vi "增加角点.vi"(9 "原始角点坐标":cluster{"X":sgl, "Y":sgl}[](array[cluster]), 11 "Image In":T1) -> (1 "原始角点坐标 2":cluster{"X":sgl, "Y":sgl}[](array[cluster]), 3 "角点图":T1(plugin-control))   [LabVIEW 2018]
uses:
  <vilib>/vision/Image Controls.llb/IMAQ Image.ctl
  <vilib>/vision/NI_Vision_Development_Module.lvlib
panel:
  in  "角点的最小强度":i32
  in  "刷新按钮":bool
  in  "快进按钮":bool
  out "Corner Point Coordinates":cluster{"X":sgl, "Y":sgl}[](array[cluster])
  out "Image (duplicate)":T1
  in  "确定按钮":bool
  in  "停止角点增加":bool
  in  "操作类型":bool
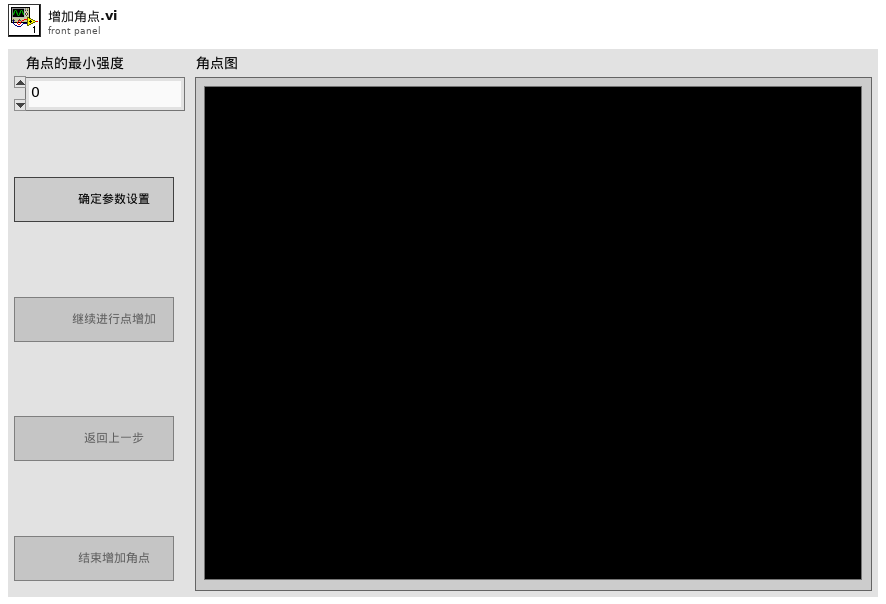
[diagram p1: front panel]
types:
  T1 = typedef "IMAQ Image.ctl" = refnum<image>
  T2 = enum8{"Enabled", "Disabled", "Disabled and Grayed Out"}
  T3 = typedef "IMAQ Rectangle" = cluster{"Left":i32, "Top":i32, "Right":i32, "Bottom":i32, "Rotation":dbl}
  T4 = typedef "ROI Descriptor" = cluster{"Global Rectangle":i32[], "Contours":cluster{"ID":enum32{"External", "Internal"}, "Type":u32, "Coordinates":i32[]}[]}
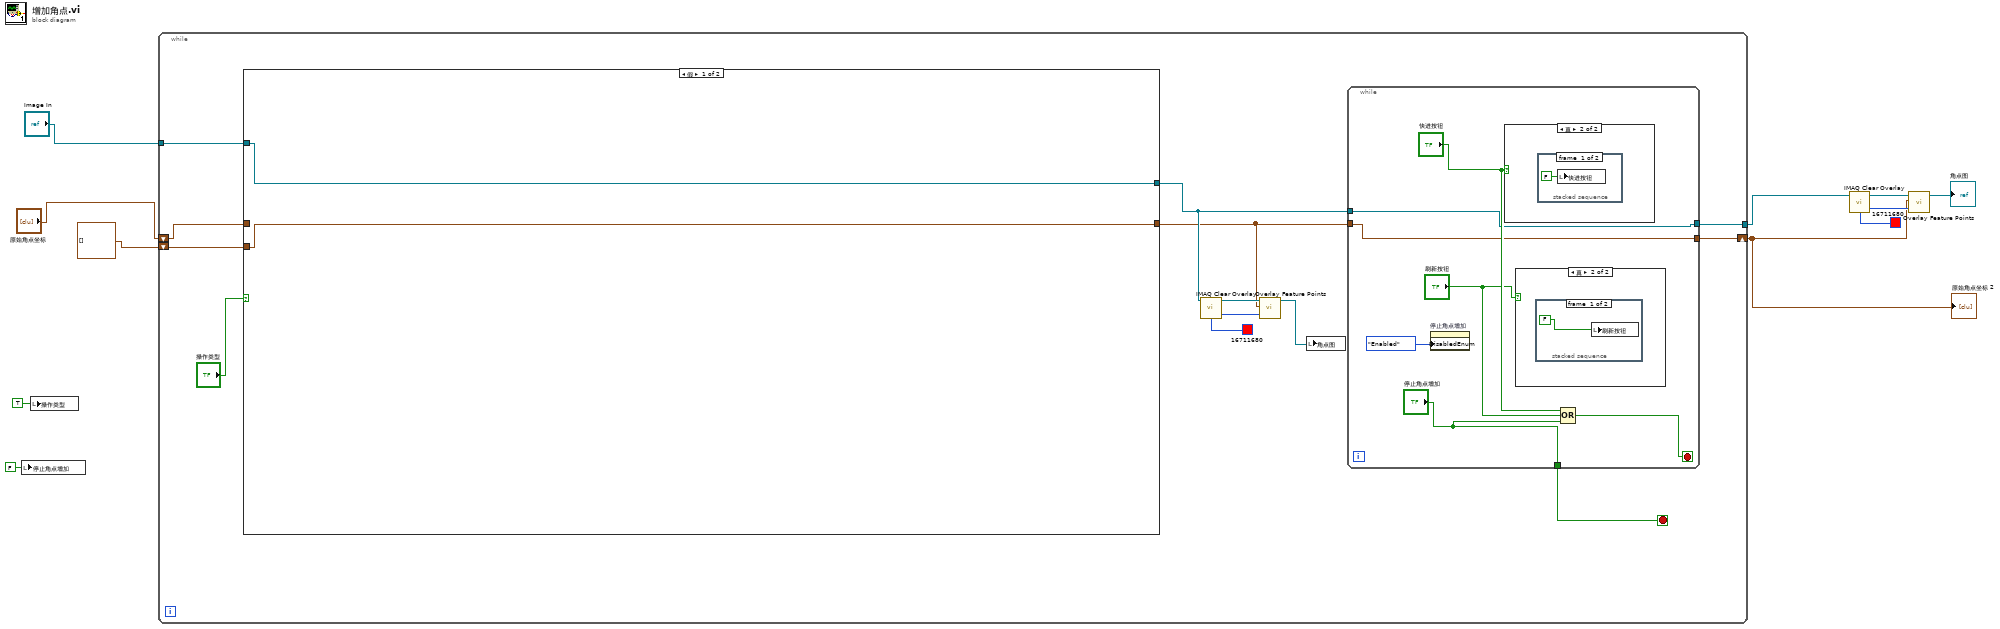
[diagram p0: block diagram]
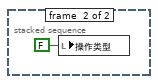
[diagram p3: hidden frame]
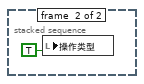
[diagram p5: hidden frame]
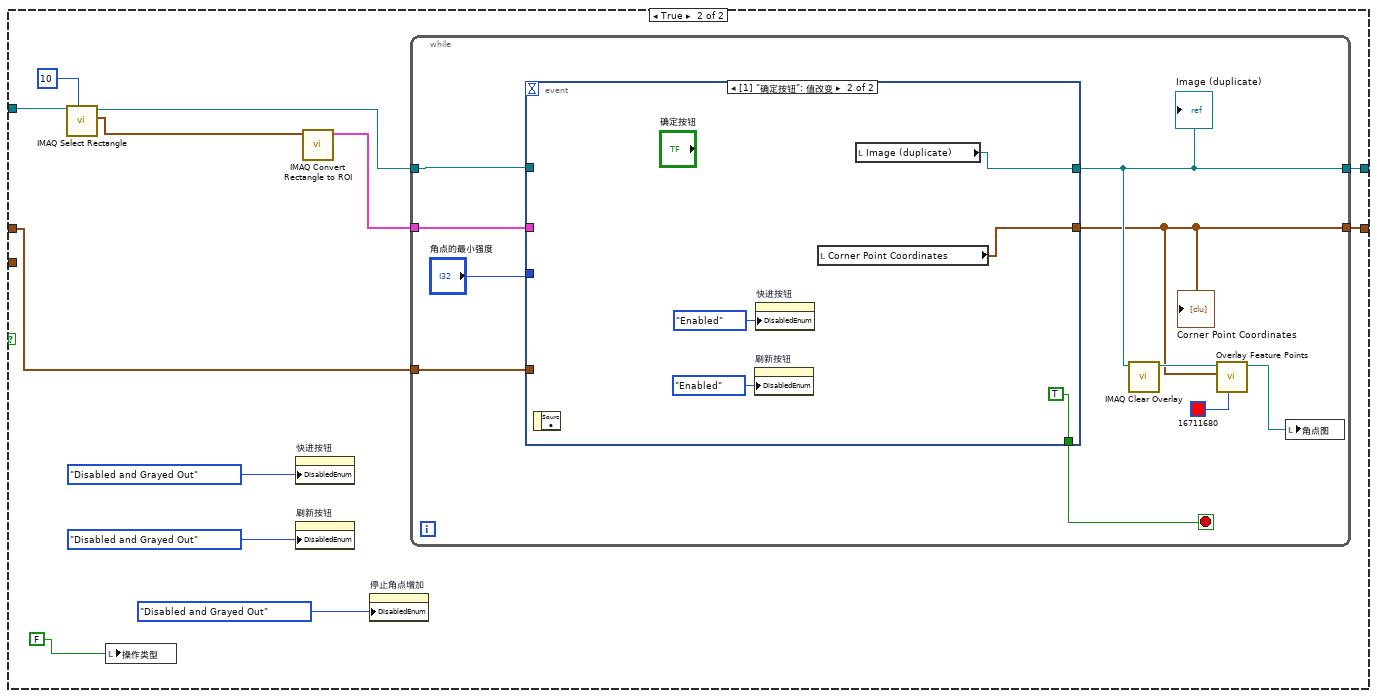
[diagram p6: hidden frame]
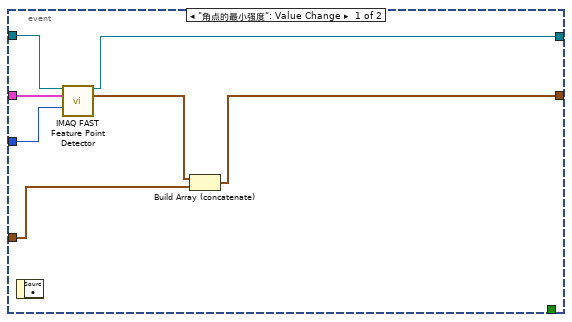
[diagram p7: hidden frame]
diagram:
  n1 = local write "停止角点增加"(FALSE ("停止角点增加")) -> ()
  n2 = local write "操作类型"(TRUE) -> ()
  n3 = while {
    shift-right: [w18] -> w8
    shift-left: "原始角点坐标" -> [w22]
    shift-left: cluster{"X":sgl, "Y":sgl}[] [] ("原始角点坐标") -> [w19]
    tunnel: "Image In" -> [w21]
    tunnel: [w16] -> w5
    stop <- w17 stop-if-true
    n4 = case shown="假" "操作类型" {
      tunnel: w22 -> [_ w39]
      tunnel: w21 -> [w35 w47]
      tunnel: [w34 w40] -> w11
      tunnel: [w35 w43] -> w12
      tunnel: w19 -> [w34 _]
      frame False {
      }
      frame True {
        n5 = call "IMAQ Select Rectangle"("Window Number (0...15)"=10, "Image In"=w47) -> ("Rectangle"=w41:T3, "Image Out (duplicate)"=w44:T1)  [unwired: 6 in, 2 out]
        n6 = local write "操作类型"(FALSE) -> ()
        n7 = property on="快进按钮" class="Bool (严格)"("DisabledEnum"=T2."Disabled and Grayed Out" ("禁用")) -> ()  [unwired: 2 in, 2 out]
        n8 = property on="刷新按钮" class="Bool (严格)"("DisabledEnum"=T2."Disabled and Grayed Out" ("禁用")) -> ()  [unwired: 2 in, 2 out]
        n9 = call "IMAQ Convert Rectangle to ROI"("Rectangle"=w41) -> ("ROI Descriptor"=w42:T4)  [unwired: 8 in, 1 out]
        n10 = property on="停止角点增加" class="Bool (严格)"("DisabledEnum"=T2."Disabled and Grayed Out" ("禁用")) -> ()  [unwired: 2 in, 2 out]
        n11 = while {
          tunnel: w42 -> [w56]
          tunnel: [w49] -> w40
          tunnel: w44 -> [w57]
          tunnel: [w50] -> w43
          tunnel: w39 -> [w54]
          stop <- w55 stop-if-true
          n12 = event shown="[1] \"确定按钮\": 值改变" {
            selector: _ -> [_ _]
            dyn-events: _ -> [_ _]
            timeout: _ -> [_ _]
            tunnel: w57 -> [w64 _]
            tunnel: w56 -> [w63 _]
            tunnel: [w59 w68] -> w49
            tunnel: [w62 w67] -> w50
            tunnel: [_ TRUE] -> w55
            tunnel: w54 -> [w61 _]
            tunnel: "角点的最小强度" -> [w58 _]
            event "角点的最小强度": Value Change {
              n13 = event-data() -> ()  [unwired: 1 in, 1 out]
              n14 = call "IMAQ FAST Feature Point Detector"("Image"=w64, "ROI Descriptor"=w63, "Min Feature Point Strength"=w58) -> ("Image (duplicate)"=w62:T1, "Feature Point Coordinates"=w60:cluster{"X":sgl, "Y":sgl}[])  [unwired: 7 in, 4 out]
              n15 = Build Array (concatenate)(w60, w61) -> (w59:cluster{"X":sgl, "Y":sgl}[])
            }
            event "确定按钮": Value Change {
              n16 = event-data() -> ()  [unwired: 1 in, 1 out]
              n17 = property on="刷新按钮" class="Bool (严格)"("DisabledEnum"=T2."Enabled" ("禁用")) -> ()  [unwired: 2 in, 2 out]
              n18 = property on="快进按钮" class="Bool (严格)"("DisabledEnum"=T2."Enabled" ("禁用")) -> ()  [unwired: 2 in, 2 out]
              n19 = local read "Corner Point Coordinates"() -> (w68:cluster{"X":sgl, "Y":sgl}[])
              n20 = local read "Image (duplicate)"() -> (w67:T1)
            }
          }
          "Image (duplicate)" <- w50
          "Corner Point Coordinates" <- w49
          n21 = call "IMAQ Clear Overlay"("Image"=w50) -> ("Image Out"=w51:T1)  [unwired: 9 in, 1 out]
          n22 = call "Overlay Feature Points.vi"("Color"=u32 16711680, "Feature Points"=w49, "Image"=w51) -> ("Image Out"=w53:T1)  [unwired: 7 in, 1 out]
          n23 = local write "角点图"(w53) -> ()
        }
      }
    }
    n24 = call "IMAQ Clear Overlay"("Image"=w12) -> ("Image Out"=w13:T1)  [unwired: 9 in, 1 out]
    n25 = call "Overlay Feature Points.vi"("Color"=u32 16711680, "Feature Points"=w11, "Image"=w13) -> ("Image Out"=w15:T1)  [unwired: 7 in, 1 out]
    n26 = local write "角点图"(w15) -> ()
    n27 = while {
      tunnel: ["停止角点增加"] -> w17
      tunnel: w11 -> [w26]
      tunnel: [w26] -> w18
      tunnel: [w24] -> w16
      tunnel: w12 -> [w24]
      stop <- w27 stop-if-true
      n28 = property on="停止角点增加" class="Bool (严格)"("DisabledEnum"=T2."Enabled" ("禁用")) -> ()  [unwired: 2 in, 2 out]
      n29 = case shown="真" "快进按钮" {
        frame False {
        }
        frame True {
          n30 = stacked-sequence {
            frame #0 {
              n31 = local write "快进按钮"(FALSE ("快进按钮")) -> ()
            }
            frame #1 {
              n32 = local write "操作类型"(TRUE) -> ()
            }
          }
        }
      }
      n33 = case shown="真" "刷新按钮" {
        frame False {
        }
        frame True {
          n34 = stacked-sequence {
            frame #0 {
              n35 = local write "刷新按钮"(FALSE) -> ()
            }
            frame #1 {
              n36 = local write "操作类型"(FALSE ("操作类型")) -> ()
            }
          }
        }
      }
      n37 = Compound Arithmetic op=OR("快进按钮", "刷新按钮", "停止角点增加") -> (w27:bool)
    }
  }
  "原始角点坐标 2" <- w8
  n38 = call "IMAQ Clear Overlay"("Image"=w5) -> ("Image Out"=w9:T1)  [unwired: 9 in, 1 out]
  n39 = call "Overlay Feature Points.vi"("Color"=u32 16711680, "Feature Points"=w8, "Image"=w9) -> ("Image Out"=→"角点图":T1)  [unwired: 7 in, 1 out]
